vi "Rotate2D.vi"(0 "x":dbl=1.0, 1 "mx":dbl, 2 "y":dbl=1.0, 3 "my":dbl, 4 "alpha(rad)":dbl) -> (5 "xout":dbl, 6 "yout":dbl)   [LabVIEW 2015]
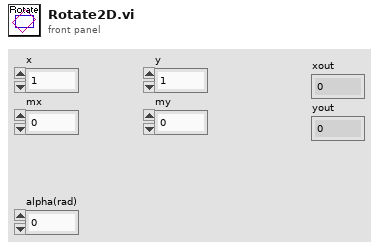
[diagram p1: front panel]
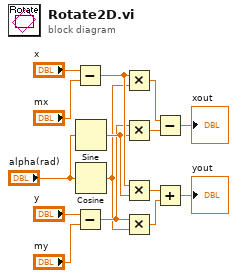
[diagram p0: block diagram]
diagram:
  n1 = Subtract(x="x", y="mx") -> (x-y=w4:dbl)
  n2 = Subtract(x="y", y="my") -> (x-y=w2:dbl)
  n3 = Sine(x="alpha(rad)") -> (sin(x)=w3:dbl)
  n4 = Cosine(x="alpha(rad)") -> (cos(x)=w1:dbl)
  n5 = Multiply(x=w4, y=w1) -> (x*y=w10:dbl)
  n6 = Multiply(x=w2, y=w3) -> (x*y=w9:dbl)
  n7 = Multiply(x=w4, y=w3) -> (x*y=w8:dbl)
  n8 = Multiply(x=w2, y=w1) -> (x*y=w7:dbl)
  n9 = Subtract(x=w10, y=w9) -> (x-y=→"xout":dbl)
  n10 = Add(x=w8, y=w7) -> (x+y=→"yout":dbl)
